vi "PLC COMMUNICATION TEST.vi"() -> ()   [LabVIEW 2017]
uses:
  <vilib>/NI/Modbus Library/API/Wrapper/Create TCP Master.vi
  <vilib>/NI/Modbus Library/API/Master/Modbus Master.lvclass
  <vilib>/NI/Modbus Library/API/Wrapper/API Main.lvlib
panel:
  in  "milliseconds to wait":u32=500
  in  "Write M":bool
  in  "Write D":bool
  out "D register write error":errorcluster
  in  "Data to \nwrite":u16[](array[numeric])
  in  "Write starting \naddress D0 = 0":u16
  out "M register Write error":errorcluster
  in  "Write starting \naddress M0 = 8192":u16=8192
  out "M register read error":errorcluster
  in  "number of inputs M":u16
  in  "Read starting \naddress M0 = 8192":u16=8192
  out "D register readerror":errorcluster
  in  "Read starting \naddress D0 = 0":u16
  in  "number of inputs":u16
  in  "address":string="192.168.3.20"
  out "error out":errorcluster
  in  "error in":errorcluster
  in  "stop":bool
  out "Read D Values":u16[](array[numeric])
  in  "Write to PLC M":bool[](array[boolean])
  out "Scanned Value D6000":string
  out "Read M Values":bool[](array[boolean])
  # "This is for Mitsubishi PLC"
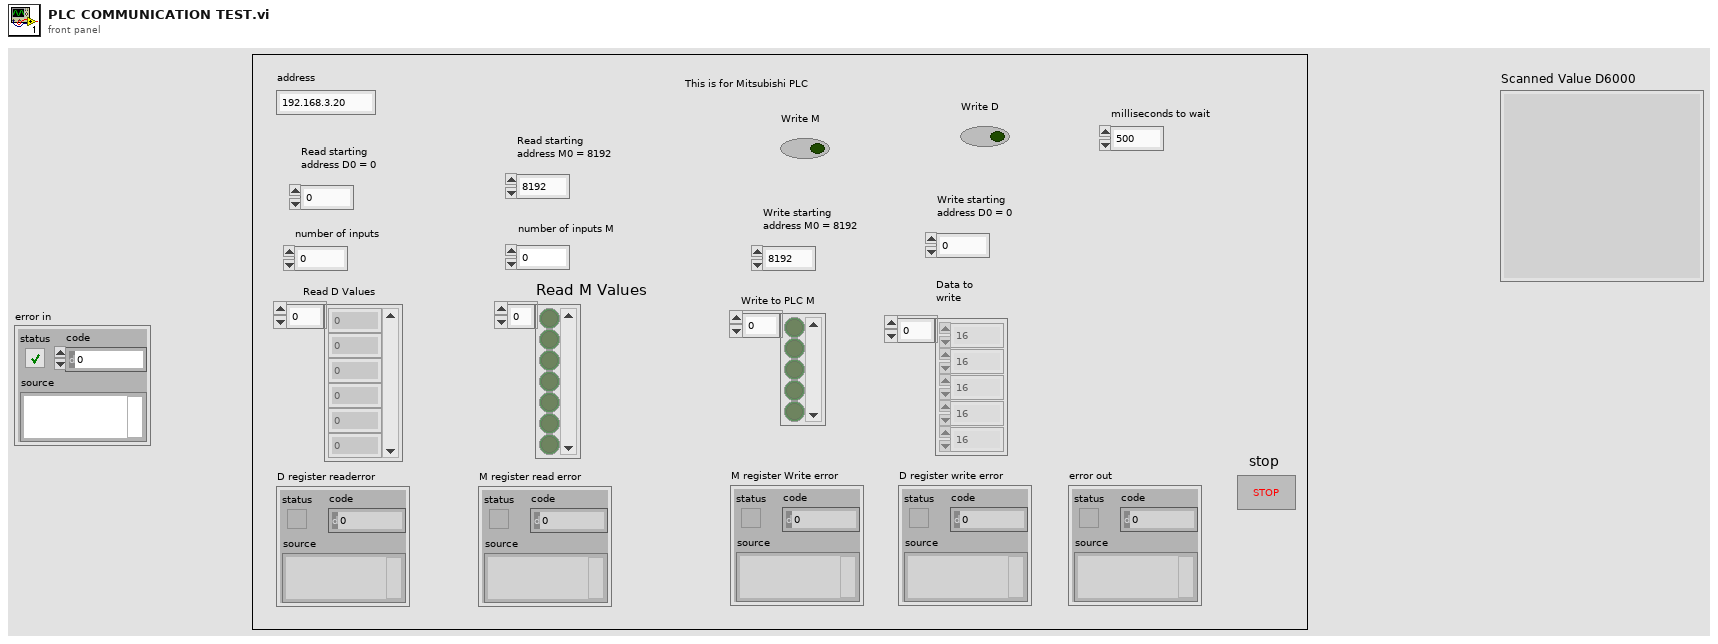
[diagram p1: front panel]
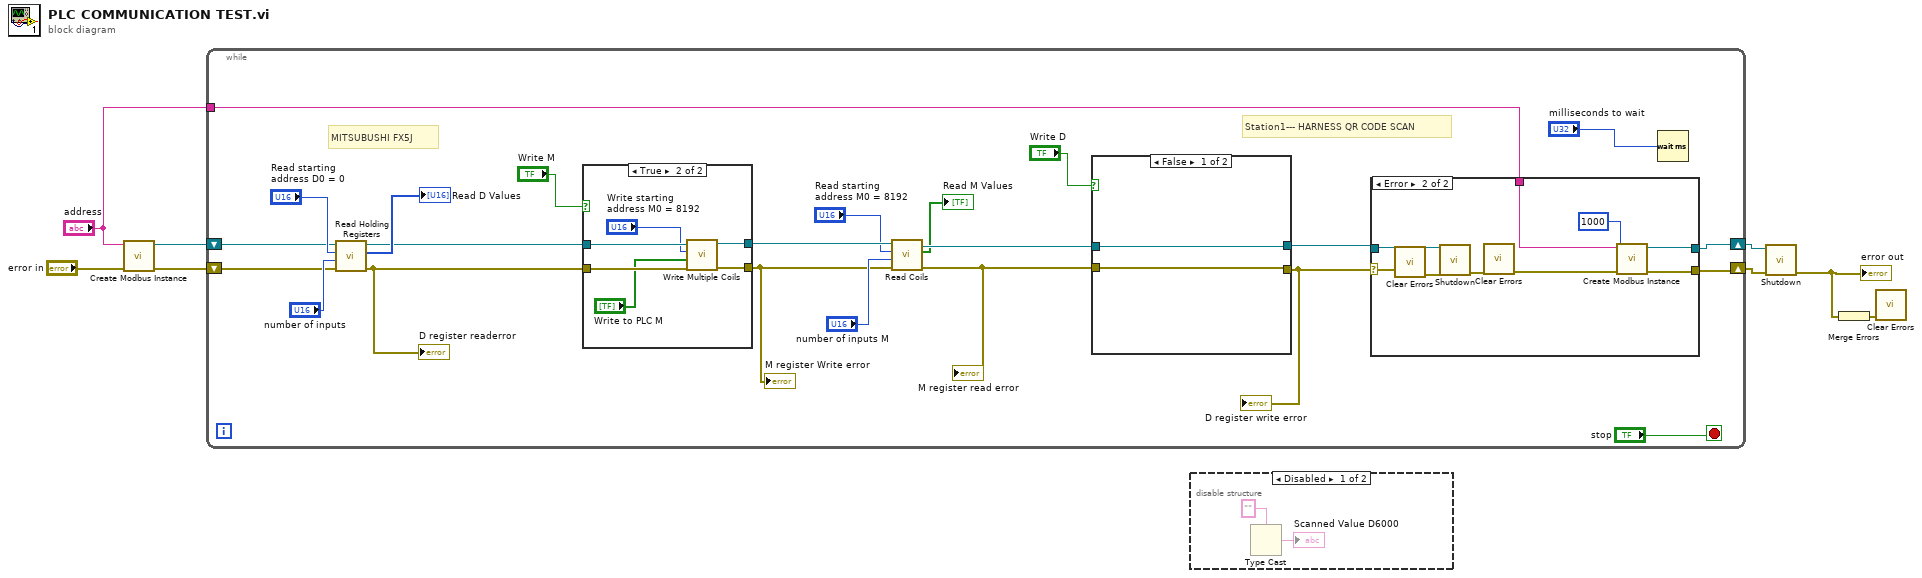
[diagram p0: block diagram]
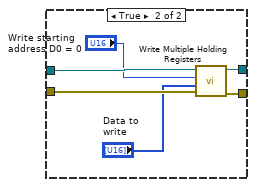
[diagram p3: hidden frame]
diagram:
  n1 = call-poly <vilib>:"Create Modbus Instance.vi"("error in"="error in", "address"="address") -> ("error out"=w6:errorcluster, "TCP master instance"=w5:refnum<class "Modbus Master.lvclass">)  [unwired: 8 in]
  n2 = while {
    shift-right: [w30] -> w8
    shift-left: w5 -> [w17]
    shift-right: [w29] -> w7
    shift-left: w6 -> [w18]
    tunnel: "address" -> [w12]
    stop <- "stop" stop-if-true
    # "Station1--- HARNESS QR CODE SCAN"
    # "MITSUBUSHI FX5J"
    n3 = call-dynamic "Read Holding Registers.vi"("error in"=w18, "number of inputs"="number of inputs", "starting address"="Read starting \naddress D0 = 0", "Modbus master in"=w17) -> ("error out"=w21:errorcluster, "register values"=→"Read D Values":u16[], "Modbus master out"=w19:refnum<class "Modbus Master.lvclass">)  [unwired: 5 in]
    "D register readerror" <- w21
    n4 = case shown="True" "Write M" {
      tunnel: [w51 w58] -> w25
      tunnel: w21 -> [w52 w57]
      tunnel: w19 -> [w51 w56]
      tunnel: [w52 w53] -> w13
      frame False {
      }
      frame True {
        n5 = call-dynamic "Write Multiple Coils.vi"("error in"=w57, "coils to write"="Write to PLC M", "starting address"="Write starting \naddress M0 = 8192", "Modbus master in"=w56) -> ("error out"=w53:errorcluster, "Modbus master out"=w58:refnum<class "Modbus Master.lvclass">)  [unwired: 6 in]
      }
    }
    "M register Write error" <- w13
    n6 = call-dynamic "Read Coils.vi"("error in"=w13, "number of inputs"="number of inputs M", "starting address"="Read starting \naddress M0 = 8192", "Modbus master in"=w25) -> ("error out"=w14:errorcluster, "coils"=→"Read M Values":bool[], "Modbus master out"=w24:refnum<class "Modbus Master.lvclass">)  [unwired: 5 in]
    "M register read error" <- w14
    n7 = case shown="False" "Write D" {
      tunnel: w24 -> [w32 w39]
      tunnel: [w32 w38] -> w23
      tunnel: w14 -> [w33 w37]
      tunnel: [w33 w35] -> w11
      frame False {
      }
      frame True {
        n8 = call-dynamic "Write Multiple Holding Registers.vi"("error in"=w37, "registers to write"="Data to \nwrite", "starting address"="Write starting \naddress D0 = 0", "Modbus master in"=w39) -> ("error out"=w35:errorcluster, "Modbus master out"=w38:refnum<class "Modbus Master.lvclass">)  [unwired: 6 in]
      }
    }
    "D register write error" <- w11
    n9 = case shown="Error" w11 {
      selector: w11 -> [w40 w50]
      tunnel: w23 -> [w41 w48]
      tunnel: [w41 w45] -> w30
      tunnel: [w40 w44] -> w29
      tunnel: w12 -> [_ w42]
      frame No Error {
      }
      frame Error {
        n10 = call <vilib>:"Clear Errors.vi"("error in (no error)"=w50) -> ("error out"=w49:errorcluster)  [unwired: 5 in, 1 out]
        n11 = call-dynamic "Shutdown.vi"("error in"=w49, "Modbus master in"=w48) -> ("error out"=w47:errorcluster)  [unwired: 9 in]
        n12 = call <vilib>:"Clear Errors.vi"("error in (no error)"=w47) -> ("error out"=w46:errorcluster)  [unwired: 5 in, 1 out]
        n13 = call-poly <vilib>:"Create Modbus Instance.vi"("error in"=w46, "connect timeout ms"=1000, "address"=w42) -> ("error out"=w44:errorcluster, "TCP master instance"=w45:refnum<class "Modbus Master.lvclass">)  [unwired: 7 in]
      }
    }
    n14 = Wait (ms)(milliseconds to wait="milliseconds to wait") -> ()  [unwired: 1 out]
  }
  n15 = disable-structure shown="Disabled" {
    frame Disabled {
      n16 = Type Cast(type="") -> (*(type *) &x=→"Scanned Value D6000":string)  [unwired: 1 in]
    }
    frame Enabled {
    }
  }
  n17 = call-dynamic "Shutdown.vi"("error in"=w7, "Modbus master in"=w8) -> ("error out"=w3:errorcluster)  [unwired: 9 in]
  "error out" <- w3
  n18 = Merge Errors(w3) -> (w2:errorcluster)
  n19 = call <vilib>:"Clear Errors.vi"("error in (no error)"=w2) -> ()  [unwired: 5 in, 2 out]
